vi "close.vi"(8 "error in":errorcluster, 11 "Engine to Engine Communication runtime in":refnum<class "E2E Runtime (RT FIFO).lvclass">) -> (0 "error out":errorcluster)   [LabVIEW 2015, in "E2E Runtime (RT FIFO).lvclass"]
doc: "Provides an interface for terminating a module instance. While this interface performs no operations, a child should close and deallocate any open references or memory."
uses:
  E2E Runtime (RT FIFO).lvclass
  E2E Runtime (RT FIFO).lvclass/E2E Runtime (RT FIFO).ctl
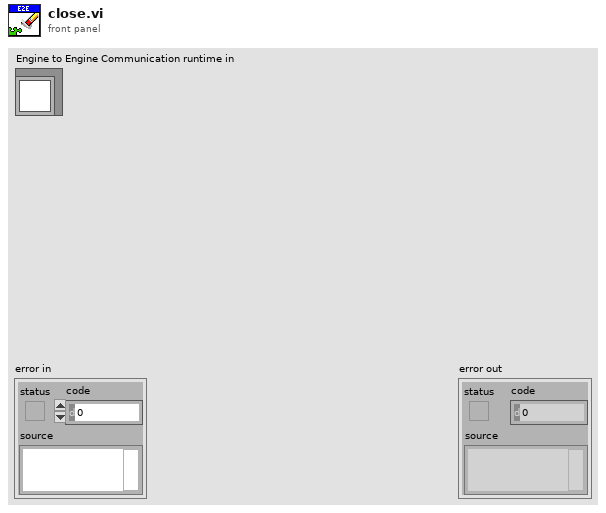
[diagram p1: front panel]
types:
  T1 = typedef "E2E Runtime (RT FIFO).lvclass/Data FIFOs.ctl" = cluster{"Double":refnum<k33>, "Single":refnum<k33>, "I64":refnum<k33>, "I32":refnum<k33>, "I16":refnum<k33>, "I8":refnum<k33>, "U64":refnum<k33>, "U32":refnum<k33>, "U16":refnum<k33>, "U8":refnum<k33>, "Boolean":refnum<k33>}
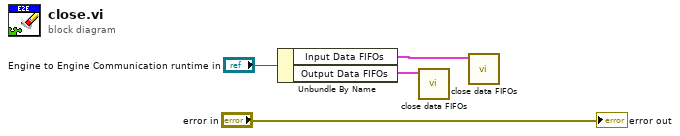
[diagram p0: block diagram]
diagram:
  n1 = Unbundle By Name("Engine to Engine Communication runtime in") -> ("Input Data FIFOs"=w2:T1, "Output Data FIFOs"=w3:T1)
  n2 = call "close data FIFOs.vi"("Data FIFOs"=w3) -> ()  [unwired: 11 in]
  n3 = call "close data FIFOs.vi"("Data FIFOs"=w2) -> ()  [unwired: 11 in]
  "error out" <- "error in"
